vi "Get Case Structure Tunnels from Shift Register.vi"(8 "error in (no error)":errorcluster, 11 "RightShiftRegister":refnum<vi>) -> (0 "error out":errorcluster, 1 "Case Structure Right Side Terminal":refnum<vi>, 2 "Case Structure Left Side Terminal":refnum<vi>)   [LabVIEW 2020, in "JKI State Machine API.lvlib" / "JKI SM.lvclass"]
uses:
  JKI SM.lvclass
  JKI SM.lvclass/JKI SM.ctl
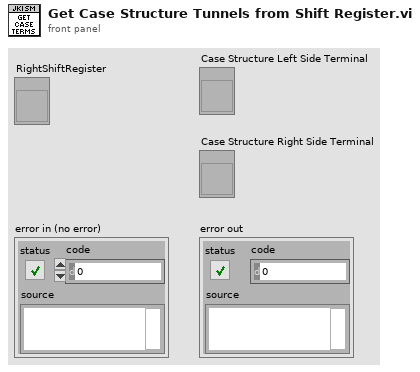
[diagram p1: front panel]
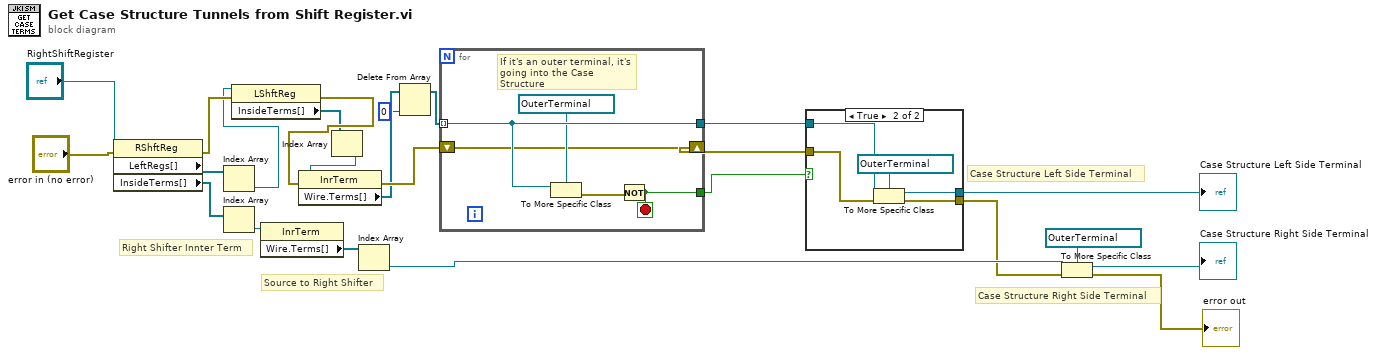
[diagram p0: block diagram]
diagram:
  # "Case Structure Left Side Terminal"
  # "Case Structure Right Side Terminal"
  # "Source to Right Shifter"
  # "Right Shifter Innter Term"
  n1 = property class="RShftReg"(reference="RightShiftRegister", error in="error in (no error)") -> (error out=w20:errorcluster, "LeftRegs[]"=w17:refnum<vi>[], "InsideTerms[]"=w21:refnum<vi>[])  [unwired: 1 out]
  n2 = Index Array(array=w17) -> (element=w18:refnum<vi>)  [unwired: 1 in]
  n3 = Index Array(array=w21) -> (element=w22:refnum<vi>)  [unwired: 1 in]
  n4 = property class="LShftReg"(reference=w18, error in=w20) -> (error out=w15:errorcluster, "InsideTerms[]"=w11:refnum<vi>[])  [unwired: 1 out]
  n5 = property class="InrTerm"(reference=w22) -> ("Wire.Terms[]"=w23:refnum<vi>[])  [unwired: 1 in, 2 out]
  n6 = Index Array(array=w11) -> (element=w12:refnum<vi>)  [unwired: 1 in]
  n7 = property class="InrTerm"(reference=w12, error in=w15) -> (error out=w13:errorcluster, "Wire.Terms[]"=w3:refnum<vi>[])  [unwired: 1 out]
  n8 = Index Array(array=w23) -> (element=w7:refnum<vi>)  [unwired: 1 in]
  n9 = Delete From Array(array=w3, index=0) -> (array with subset deleted=w1:refnum<vi>[])  [unwired: 1 in, 1 out]
  n10 = for {
    tunnel: w1 -> [w29] mode=indexing
    shift-right: [w26] -> w9
    shift-left: w13 -> [w26]
    tunnel: [w25] -> w10
    tunnel: [w29] -> w14
    stop <- w25 stop-if-true
    # "If it's an outer terminal, it's going into the Case Structure"
    n11 = To More Specific Class(target class=refnum<vi> refnum ("Part References.Case Structure"), reference=w29) -> (error out=w27:errorcluster)  [unwired: 1 in, 1 out]
    n12 = Not(x=w27) -> (.not. x?=w25:bool)
  }
  n13 = case shown="True" w10 {
    tunnel: [_ w33] -> w24
    tunnel: w14 -> [_ w35]
    tunnel: w9 -> [w30 w32]
    tunnel: [w30 w31] -> w5
    frame False {
    }
    frame True {
      n14 = To More Specific Class(target class=refnum<vi> refnum ("f"), reference=w35, error in=w32) -> (specific class reference=w33:refnum<vi>, error out=w31:errorcluster)
    }
  }
  "Case Structure Left Side Terminal" <- w24
  n15 = To More Specific Class(target class=refnum<vi> refnum ("f"), reference=w7, error in=w5) -> (specific class reference=→"Case Structure Right Side Terminal":refnum<vi>, error out=→"error out":errorcluster)
